vi "Write Child Actor Attributes.vi"(10 "Child Actor Attributes":T1, 11 "Actor in":refnum<class "Actor.lvclass">) -> (3 "Actor out":refnum<class "Actor.lvclass">)   [LabVIEW 2020, in "jettl.lvlib" / "Actor.lvclass"]
uses:
  Actor.lvclass
  Msg/Msg.lvclass
  Msg Input/Msg Input.lvclass
  Msg Output/Msg Output.lvclass
  Child Actor Attributes.ctl
  jettl.lvlib
  Actor Attributes.ctl
  Msgs.ctl
  Unified Layer.ctl
  Relation.ctl
  Teller.ctl
  Msg Attributes.ctl
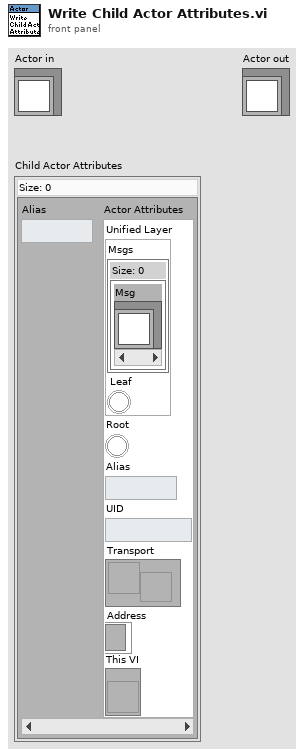
[diagram p1: front panel]
types:
  T1 = typedef "jettl.lvlib/Child Actor Attributes.ctl" = map{string, T2}
  T2 = typedef "jettl.lvlib/Actor Attributes.ctl" = cluster{"Unified Layer":T3, "Root":bool, "Alias":string, "UID":i32, "Transport":refnum<user-event>, "Address":refnum<event-registration>, "This VI":refnum<vi>}
  T3 = typedef "jettl.lvlib/Unified Layer.ctl" = cluster{"Msgs":T4, "Leaf":bool}
  T4 = typedef "jettl.lvlib/Msgs.ctl" = set{refnum<class "Msg.lvclass">}
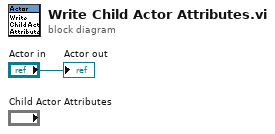
[diagram p0: block diagram]
diagram:
  "Actor out" <- "Actor in"
